vi "Sandbox.vi"() -> ()   [LabVIEW 2019]
uses:
  8d4a871f-ea0f-4aa7-a547-4d24cb021f7c.vi
  <vilib>/gpm_packages/@cs/event-logger/Source/Composed Log/LoggerReference/LoggerReference.lvclass
  7cb621b1-baf2-4cf0-84d6-a805fdf9e794.vi
  <vilib>/gpm_packages/@cs/event-logger/Source/String Control Sink/String Control Sink.lvclass
  <vilib>/gpm_packages/@cs/Network-interface/Source/Network Messenger/Network Messenger.lvclass
  cbdfa282-940e-4c4d-bd65-94c429f3b630.vi
  <vilib>/Analysis/NI_AALBase.lvlib
  <vilib>/Analysis/baseanly.llb/Mean (DBL).vi
  <vilib>/gpm_packages/@cs/Network-interface/Source/Network Messenger/IPacket Return/IPacket Return.lvclass
panel:
  out "error out":errorcluster
  out "Array":dbl[](array[numeric])
  out "min value":dbl
  out "max value":dbl
  out "mean":dbl format="%0.6f"
  out "Cycle Time":dbl
  out "Msg":string
  in  "String":string
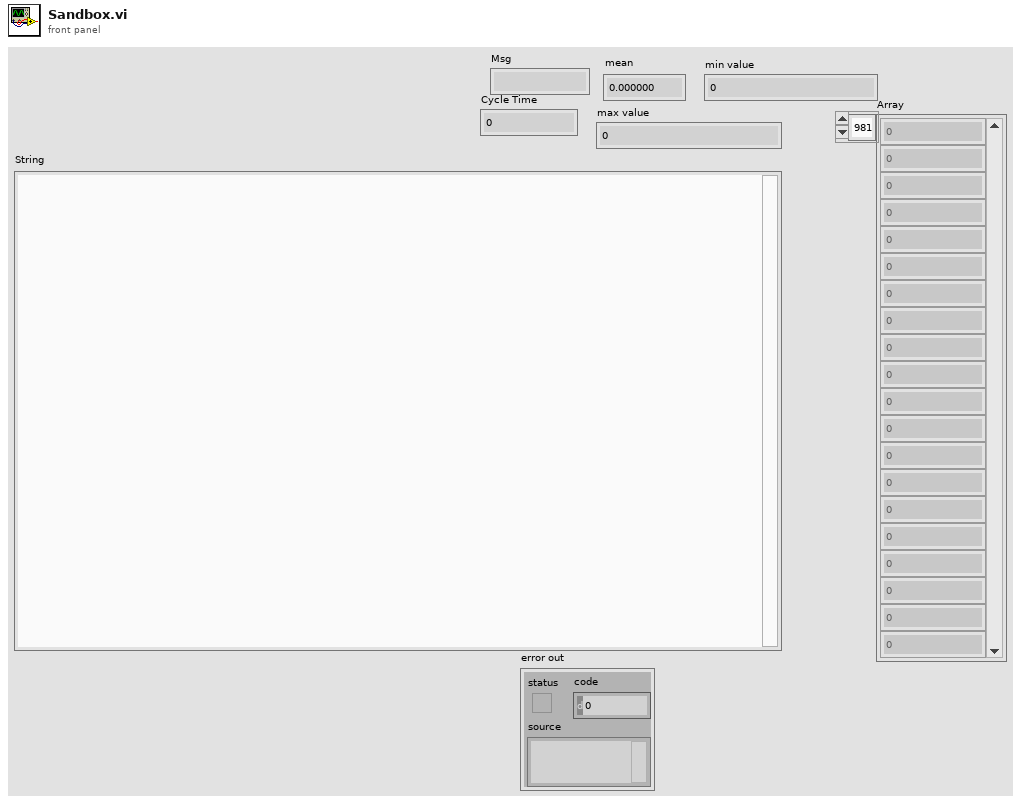
[diagram p1: front panel]
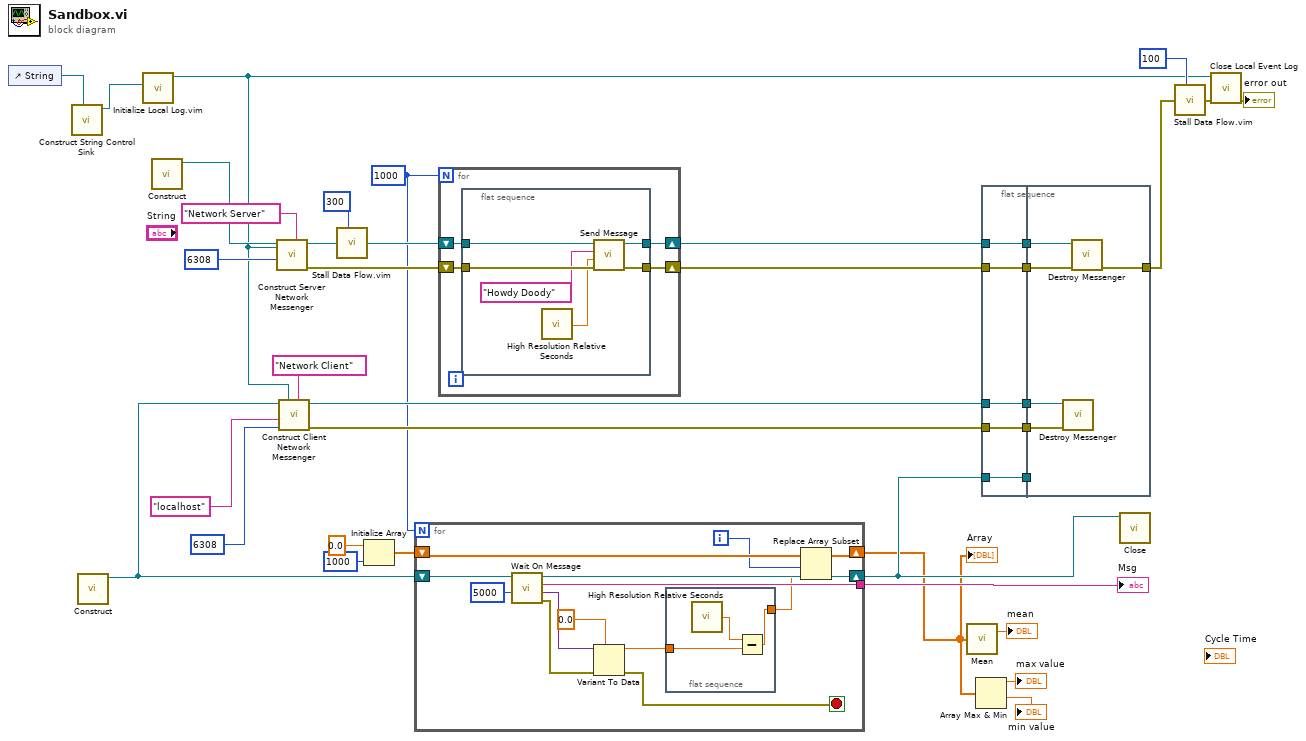
[diagram p0: block diagram]
diagram:
  w15 = 1000
  n1 = control-ref of="String"() -> (w34:refnum<vi>)
  n2 = call <vilib>:"Construct String Control Sink.vi"("Str Refnum"=w34) -> ("String Control Sink out"=w35:refnum<class "String Control Sink.lvclass">)  [unwired: 10 in]
  n3 = call <vilib>:"Construct.vi"() -> ("QueuePacketReturn out"=w25:refnum<class "QueuePacketReturn.lvclass">)  [unwired: 10 in, 1 out]
  n4 = call "Initialize Local Log.vim"("Startup Sink(s)"=w35) -> ("Log Instance Reference"=w6:refnum<class "LoggerReference.lvclass">)  [unwired: 8 in, 2 out]
  n5 = call <vilib>:"Construct.vi"() -> ("QueuePacketReturn out"=w29:refnum<class "QueuePacketReturn.lvclass">)  [unwired: 10 in, 1 out]
  n6 = call <vilib>:"Construct Server Network Messenger.vi"("Log Alias"="Network Server", "Log Instance"=w6, "Port"=u16 6308, "Packet Return"=w29) -> ("error out"=w31:errorcluster, "Network Node"=w32:refnum<data-value>)  [unwired: 6 in]
  n7 = call <vilib>:"Construct Client Network Messenger.vi"("Log Alias"="Network Client", "Log Instance"=w6, "Remote Port or Service Name"=u16 6308, "Remote IP"="localhost", "Packet Return"=w25) -> ("error out"=w21:errorcluster, "Network Node"=w22:refnum<data-value>)  [unwired: 5 in]
  n8 = call "Stall Data Flow.vim"("value in"=w32, "milliseconds to wait"=u32 300) -> ("value out"=w19:refnum<data-value>)  [unwired: 1 out]
  n9 = Initialize Array(0.0 ("element"), 1000 ("dimension size")) -> (w9:dbl[])
  n10 = for {
    N: w15 -> [_]
    tunnel: [w49] -> w24
    shift-right: [w47] -> w23
    shift-left: w25 -> [w50]
    shift-right: [w43] -> w8
    shift-left: w9 -> [w42]
    i -> [w40]
    stop <- w38 stop-if-true
    n11 = call <vilib>:"Wait On Message.vi"("timeout in ms (-1)"=5000, "QueuePacketReturn in"=w50) -> ("error out"=w39:errorcluster, "Data"=w46:variant, "Msg"=w49:string, "QueuePacketReturn out"=w47:refnum<class "QueuePacketReturn.lvclass">)  [unwired: 5 in, 1 out]
    n12 = Variant To Data(error in=w39, type=0.0, Variant=w46) -> (data=w44:dbl, error out=w38:errorcluster)
    n13 = flat-sequence {
      tunnel: [w52] -> w41
      tunnel: w44 -> [w51]
      frame #0 {
        n14 = call <vilib>:"High Resolution Relative Seconds.vi"() -> ("relative seconds"=w53:dbl)
        n15 = Subtract(x=w53, y=w51) -> (x-y=w52:dbl)
      }
    }
    n16 = Replace Array Subset(array=w42, new element=w41, index=w40) -> (w43:dbl[])
  }
  "Msg" <- w24
  "Array" <- w8
  n17 = for {
    N: w15 -> [_]
    shift-right: [w55] -> w30
    shift-left: w31 -> [w56]
    shift-right: [w57] -> w33
    shift-left: w19 -> [w54]
    n18 = flat-sequence {
      tunnel: [w63] -> w57
      tunnel: w56 -> [w62]
      tunnel: [w61] -> w55
      tunnel: w54 -> [w59]
      frame #0 {
        n19 = call <vilib>:"High Resolution Relative Seconds.vi"() -> ("relative seconds"=w58:dbl)
        n20 = call <vilib>:"Send Message.vi"("error in (no error)"=w62, "Data"=w58, "Message"="Howdy Doody", "Persistant Network Node In"=w59) -> ("error out"=w61:errorcluster, "Persistant Network Node Out"=w63:refnum<data-value>)  [unwired: 6 in]
      }
    }
  }
  n21 = call-poly <vilib>:"Mean.vi"("X"=w8) -> ("mean"=→"mean":dbl)  [unwired: 1 out]
  n22 = Array Max & Min(array=w8) -> (max value=→"max value":dbl, min value=→"min value":dbl)  [unwired: 2 out]
  n23 = flat-sequence {
    tunnel: w21 -> [w64]
    tunnel: w22 -> [w65]
    tunnel: w23 -> [w66]
    tunnel: w30 -> [w67]
    tunnel: w33 -> [w68]
    tunnel: [w68] -> w5
    tunnel: [w67] -> w4
    tunnel: [w66] -> w3
    tunnel: [w65] -> w2
    tunnel: [w64] -> w1
    tunnel: [w69] -> w20
    tunnel: w5 -> [w73]
    tunnel: w4 -> [w72]
    tunnel: w3 -> [_]
    tunnel: w2 -> [w71]
    tunnel: w1 -> [w70]
    frame #0 {
    }
    frame #1 {
      n24 = call <vilib>:"Destroy Messenger.vi"("error in (no error)"=w70, "Network Client Reference In"=w71) -> ()  [unwired: 9 in, 1 out]
      n25 = call <vilib>:"Destroy Messenger.vi"("error in (no error)"=w72, "Network Client Reference In"=w73) -> ("error out"=w69:errorcluster)  [unwired: 9 in]
    }
  }
  n26 = call <vilib>:"Close.vi"("QueuePacketReturn in"=w23) -> ()  [unwired: 10 in, 1 out]
  n27 = call "Stall Data Flow.vim"("value in"=w20, "milliseconds to wait"=u32 100) -> ("value out"=w37:errorcluster)  [unwired: 1 out]
  n28 = call <vilib>:"Close Local Event Log.vi"("error in (no error)"=w37, "Log Instance"=w6) -> ("error out"=→"error out":errorcluster)  [unwired: 9 in]
